vi "Load Formula Aliases.vi"(8 "error in (no error)":errorcluster, 11 "Dialog? (F)":bool) -> (0 "error out":errorcluster, 1 "Descriptions Array":string[](array[string]), 2 "Definitions Array":string[](array[string]), 3 "Aliases Array":string[](array[string]), 4 "Cancelled/Error":bool, 5 "File Content":string[](array[string]))   [LabVIEW 2021, in "Formula.lvlib"]
uses:
  Formula.lvlib
  <userlib>/_OpenG.lib/string/string.llb/openg_string.lvlib
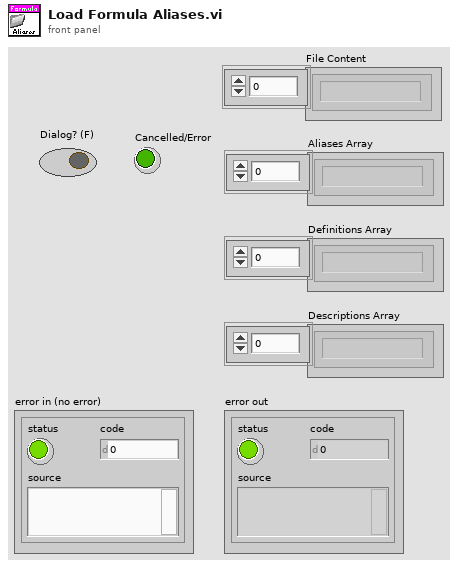
[diagram p1: front panel]
types:
  T1 = enum16{"open", "replace", "create", "open or create", "replace or create", "replace or create with confirmation"}
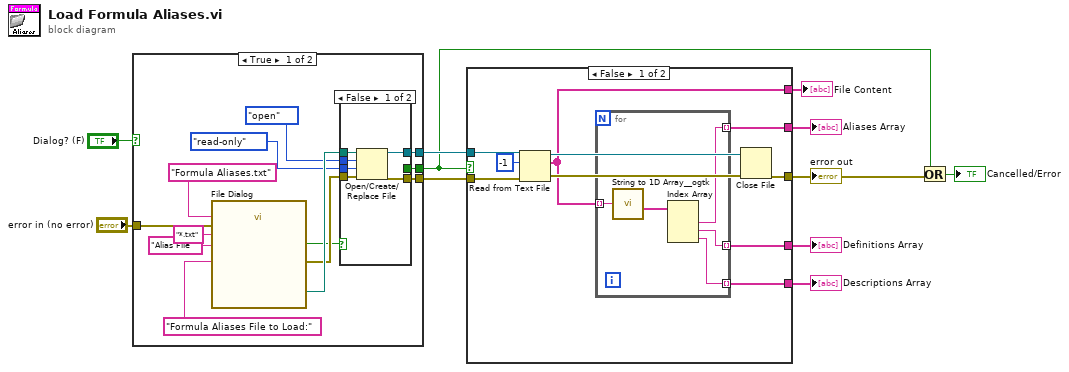
[diagram p0: block diagram]
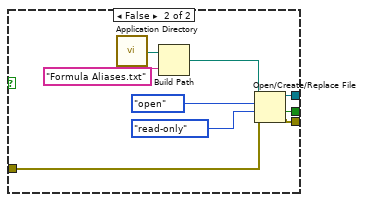
[diagram p3: hidden frame]
diagram:
  n1 = case shown="True" "Dialog? (F)" {
    tunnel: [w15 w39] -> w8
    tunnel: "error in (no error)" -> [w24 w38]
    tunnel: [w14 w37] -> w6
    tunnel: [w12 w36] -> w4
    frame True {
      n2 = call "File Dialog"("prompt"="Formula Aliases File to Load:", "default name"="Formula Aliases.txt" ("name or relative path"), "error in"=w24, "pattern (all files)"="*.txt", "pattern label"="Alias File") -> ("selected path"=w19:path, "cancelled"=w13:bool, "error out"=w16:errorcluster)  [unwired: 7 in, 1 out]
      n3 = case shown="False" w13 {
        selector: w13 -> [_ w31]
        tunnel: w19 -> [w30 _]
        tunnel: T1."open" ("operation (0:open)") -> [w29 _]
        tunnel: enum16{"read/write", "read-only", "write-only"}."read-only" ("access (0:read/write)") -> [w28 _]
        tunnel: w16 -> [w27 w32]
        tunnel: [w26 _] -> w15
        tunnel: [w25 w32] -> w14
        tunnel: [_ w31] -> w12
        frame False {
          n4 = Open/Create/Replace File(file path (use dialog)=w30, error in=w27, operation (0:open)=w29, access (0:read/write)=w28) -> (refnum out=w26:refnum<file>, error out=w25:errorcluster)  [unwired: 2 in, 1 out]
        }
        frame True {
        }
      }
    }
    frame False {
      n5 = call <vilib>:"Application Directory.vi"() -> ("Application Directory"=w35:path)
      n6 = Build Path(base path=w35, name or relative path="Formula Aliases.txt") -> (appended path=w34:path)
      n7 = Open/Create/Replace File(file path (use dialog)=w34, error in=w38, operation (0:open)=T1."open", access (0:read/write)=enum16{"read/write", "read-only", "write-only"}."read-only") -> (refnum out=w39:refnum<file>, cancelled=w36:bool, error out=w37:errorcluster)  [unwired: 2 in]
    }
  }
  n8 = case shown="False" w4 {
    tunnel: [w51 _] -> w11
    tunnel: [w49 _] -> w10
    tunnel: [w48 _] -> w9
    tunnel: [w47 w57] -> w5
    tunnel: w8 -> [w44 _]
    tunnel: w6 -> [w43 w57]
    tunnel: [w42 _] -> w1
    frame False {
      n9 = Read from Text File(file (use dialog)=w44, count=-1, error in=w43) -> (refnum out=w45:refnum<file>, text=w42:string[], error out=w46:errorcluster)  [unwired: 1 in, 1 out]
      n10 = for {
        tunnel: w42 -> [w56] mode=indexing
        tunnel: [w54] -> w48 mode=indexing
        tunnel: [w53] -> w49 mode=indexing
        tunnel: [w52] -> w51 mode=indexing
        n11 = call <userlib>:"String to 1D Array__ogtk.vi"("string"=w56) -> ("Array of Strings"=w55:string[])  [unwired: 10 in]
        n12 = Index Array(array=w55) -> (element #1=w54:string, element #2=w53:string, element #3=w52:string)  [unwired: 3 in]
      }
      n13 = Close File(refnum=w45, error in=w46) -> (error out=w47:errorcluster)  [unwired: 1 out]
    }
    frame True {
    }
  }
  "Descriptions Array" <- w11
  "Definitions Array" <- w10
  "Aliases Array" <- w9
  "error out" <- w5
  "File Content" <- w1
  n14 = Or(x=w4, y=w5) -> (x .or. y?=→"Cancelled/Error":bool)
